vi "Get Tag List.vi"(7 "Database Connection":refnum<k7>, 8 "Error In":errorcluster, 11 "DeviceName":string) -> (0 "Error Out":errorcluster, 3 "Tag List":string[][](array[string]))   [LabVIEW 2019]
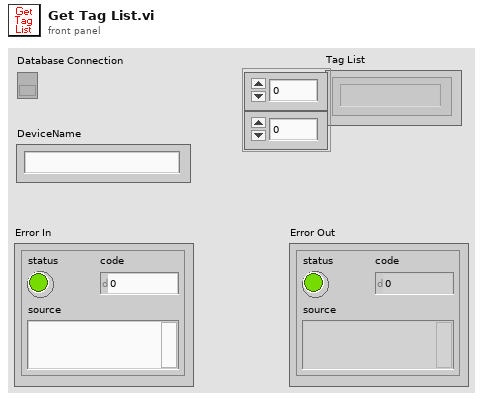
[diagram p1: front panel]
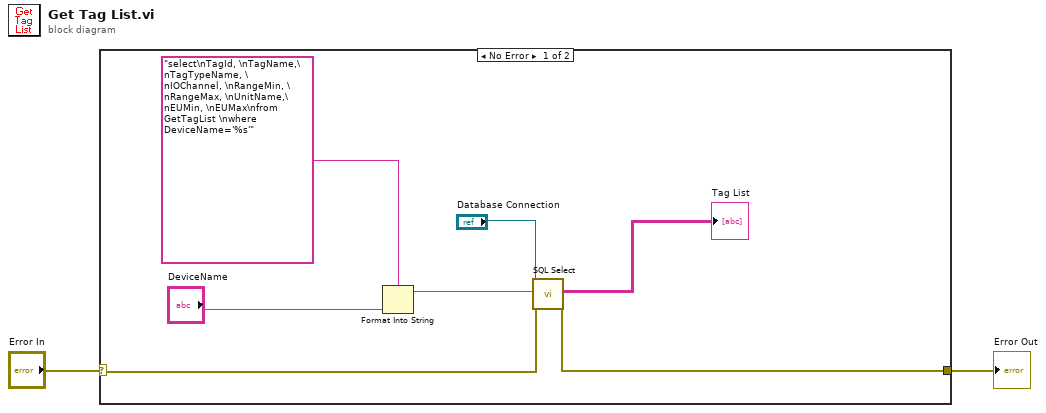
[diagram p0: block diagram]
diagram:
  n1 = case shown="No Error" "Error In" {
    selector: "Error In" -> [w8 w10]
    tunnel: [w7 w10] -> w1
    frame No Error {
      n2 = Format Into String(format string="select\nTagId, \nTagName,\nTagTypeName, \nIOChannel, \nRangeMin, \nRangeMax, \nUnitName,\nEUMin, \nEUMax\nfrom GetTagList \nwhere DeviceName='%s'", "DeviceName") -> (resulting string=w3:string)  [unwired: 2 in, 1 out]
      n3 = call <vilib>:"SQL Select.vi"("Connection In"="Database Connection", "SQL Query"=w3, "Error in (no error)"=w8) -> ("Data"=→"Tag List":string[][], "Error out"=w7:errorcluster)  [unwired: 14 in, 1 out]
    }
    frame Error {
    }
  }
  "Error Out" <- w1
